vi "CreateClass.vi"(0 "ClassWriterNative":refnum<class "ClassWriterNative.lvclass">, 1 "ProjectTreePosition(String or Project Item Ref)":variant, 2 "CreateClassData":T1, 5 "error in (no error)":errorcluster, 6 "KeepLvClassRefOpen(False)":bool, 7 "HeaderToApply (take from VIRef or /use 2D-8bit header, Ignored if not wired)":variant) -> (14 "ClassWriterNative":refnum<class "ClassWriterNative.lvclass">, 15 "LVClassLibraryRefnum":refnum<vi>, 16 "TemplateVersionUsed":string, 19 "error out":errorcluster)   [LabVIEW 2012, in "ClassWriterNative.lvclass"]
uses:
  <resource>/Framework/Providers/Open_GDS/ClassProviders/Provider_LvNativeClass/ClassWriterNative_class/ClassWriterNative.lvclass
  <resource>/Framework/Providers/Open_GDS/ClassProviders/Provider_BaseClassInterface/CreateClassData.ctl
  <resource>/Framework/Providers/Open_GDS/ClassProviders/Provider_LvNativeClass/LvNativeProviderName.ctl
  <resource>/Framework/Providers/Open_GDS/ClassProviders/Provider_LvNativeClass/Templates/LvNativeTemplateNames.ctl
  <vilib>/Utility/miscctls.llb/LVPositionTypeDef.ctl
  <resource>/Framework/Providers/Open_GDS/ClassProviders/Common/LvClass_class/GDSLvCLass_ClassSettingsType.ctl
  <resource>/Framework/Providers/Open_GDS/ClassProviders/Common/LvClass_class/GDSLvClass_PlugIn.ctl
  <resource>/Framework/Providers/Open_GDS/ClassProviders/Common/LvClass_class/GDSLvClass_PlugInTypes.ctl
  <resource>/Framework/Providers/Open_GDS/ClassProviders/Provider_BaseClassInterface/ClassWriter_class/ClassWriter.lvclass
  <vilib>/Utility/lvfile.llb/NI_FileType.lvlib
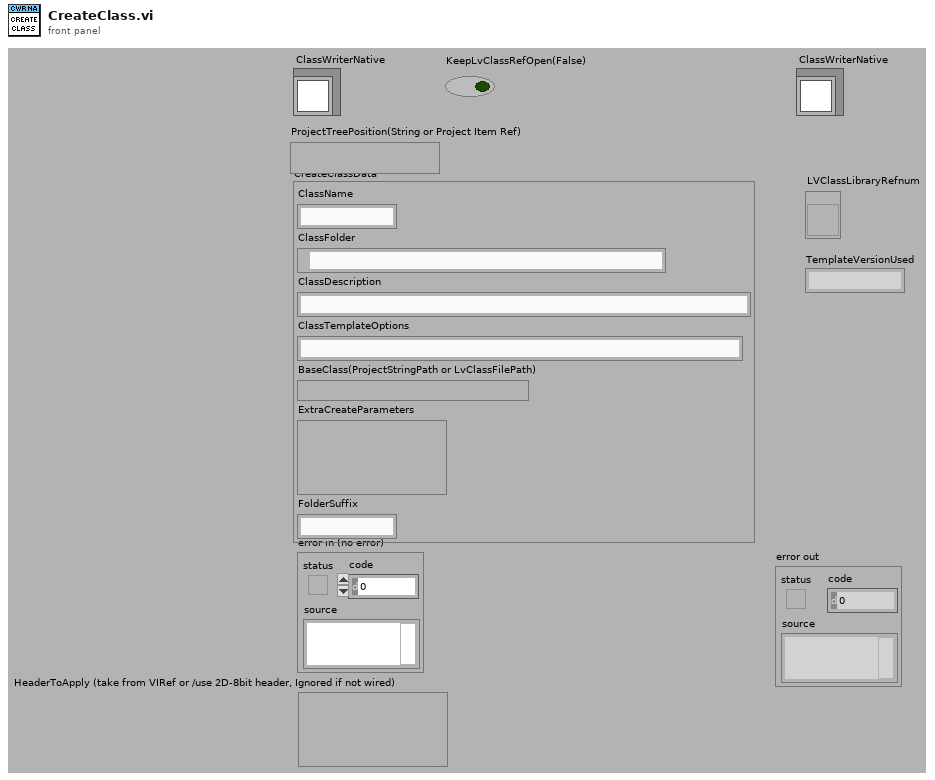
[diagram p1: front panel]
types:
  T1 = typedef "ClassWriter.lvclass/CreateClassData.ctl" = cluster{"ClassName":string, "ClassFolder":path, "ClassDescription":string, "ClassTemplateOptions":string, "BaseClass(ProjectStringPath or LvClassFilePath)":variant, "ExtraCreateParameters":variant, "FolderSuffix":string}
  T2 = cluster{"SubClass":bool, "ClassTemplateFiles":path[], "ClassName":string, "ClassFolder":path, "VIs":refnum<vi>[], "TemplateFolder":path, "ViSubDirs":string[], "TemplateName":string, "BaseClassFolder":path, "RootBaseClassFolder":path, "TemplateClass":refnum<vi>, "LvClassPath":path, "ClassRefnum":refnum<vi>, "ProjectRefnum":refnum<vi>, "LvClassFolderPath":path, "BaseClassName":string, "TemplateVersionUsed":string, "App":refnum<vi>}
  T3 = typedef "LvNativeProviderName.ctl" = enum16{"Endevo LabVIEW Native"}
  T4 = enum32{"invalid scope", "public", "private", "protected"}
  T5 = typedef "LVPositionTypeDef.ctl" = cluster{"Left":i32, "Top":i32}
  T6 = typedef "LvNativeTemplateNames.ctl" = enum16{"NativeBaseTemplate", "NativeSubTemplate", "NativeBaseTemplate_4x4x4", "NativeSubTemplate_4x4x4"}
  T7 = typedef "GDSLvCLass_ClassSettingsType.ctl" = cluster{"ClassProviderName":string, "ClassTemplateUsed":string, "ClassTemplateVersion":string, "ClassDescription":string, "PlugIns":T8[], "ConnectorPanePattern":string}
  T8 = typedef "GDSLvClass_PlugIn.ctl" = cluster{"Type":T9, "ID":string, "Version":string, "Path":path, "Name":string, "Data":variant}
  T9 = typedef "GDSLvClass_PlugInTypes.ctl" = enum16{"DesignPattern", "MethodTypes"}
  T10 = typedef "ClassWriter.lvclass/TemplateSettings.ctl" = cluster{"CommonClassTemplate":bool, "DynamicDispatch":enum8{"False", "True", "Mixed"}, "MustOverride":enum8{"False", "True", "Mixed"}, "MustCallParent":enum8{"False", "True", "Mixed"}, "OnlyNormalMethod":bool, "OnlyPublic":bool}
  T11 = typedef "Scripting_ConnectorPanePatternType.ctl" = u16
  T12 = cluster{"Major":u16, "Minor":u16, "Fix":u16, "Build":u16}
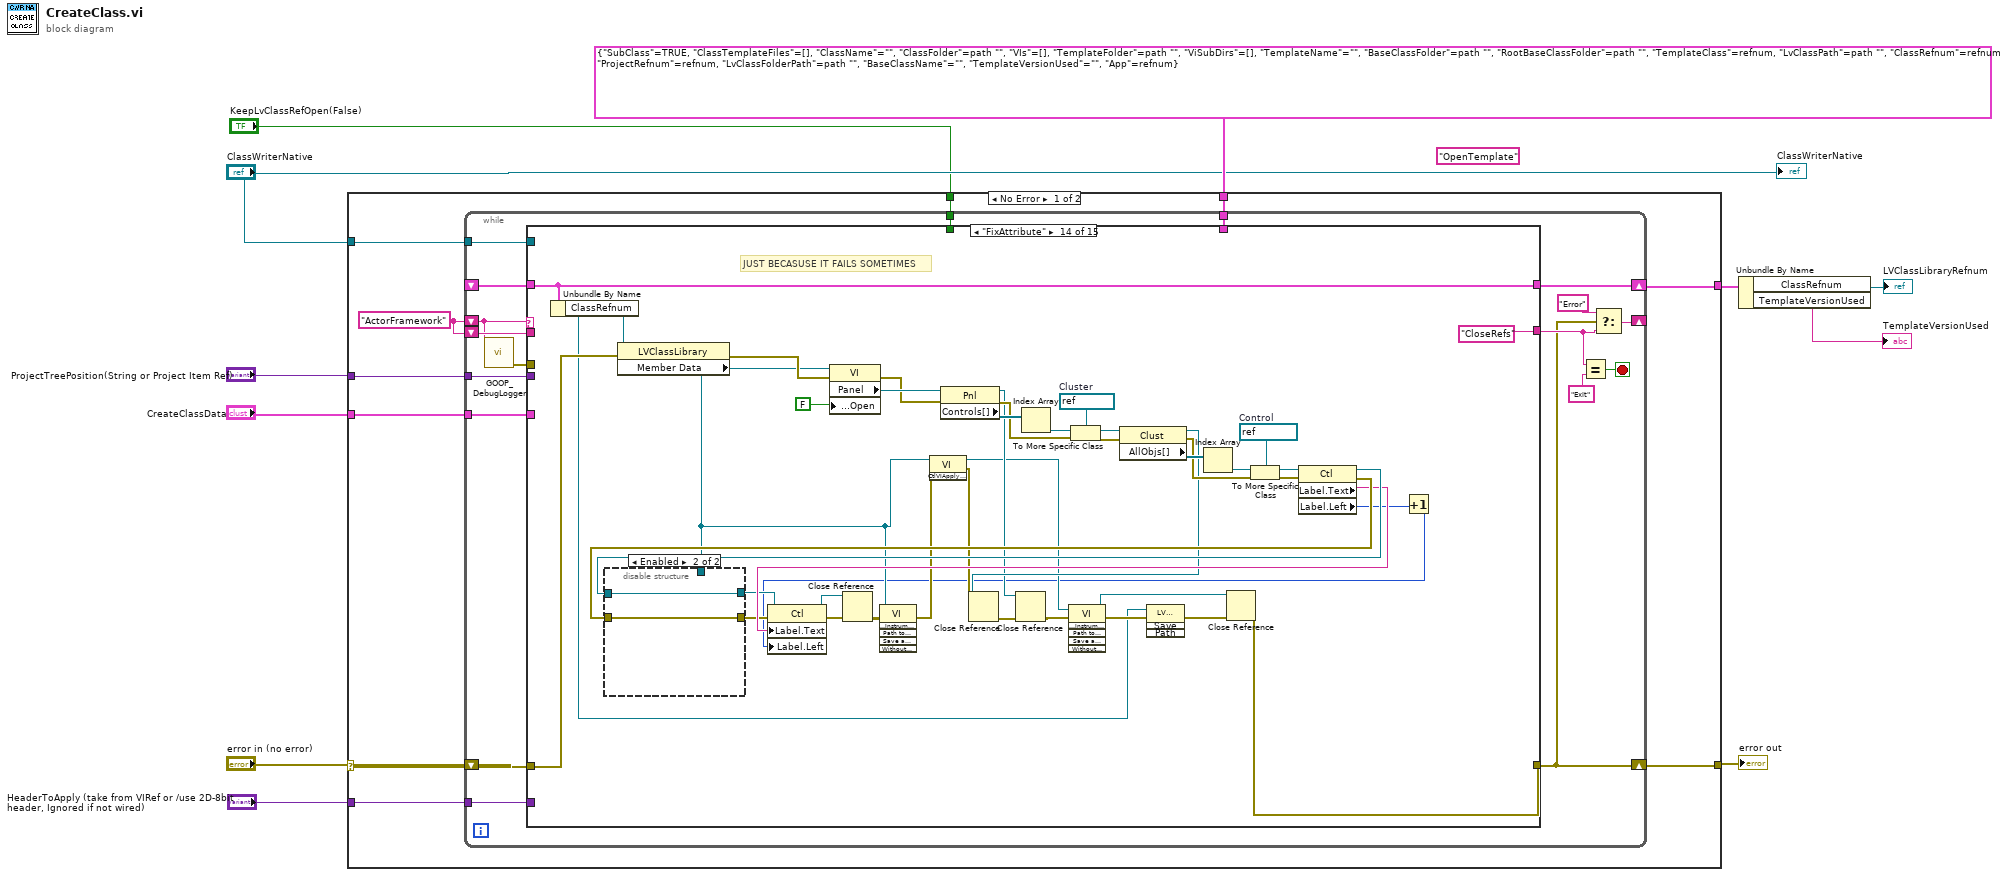
[diagram p0: block diagram]
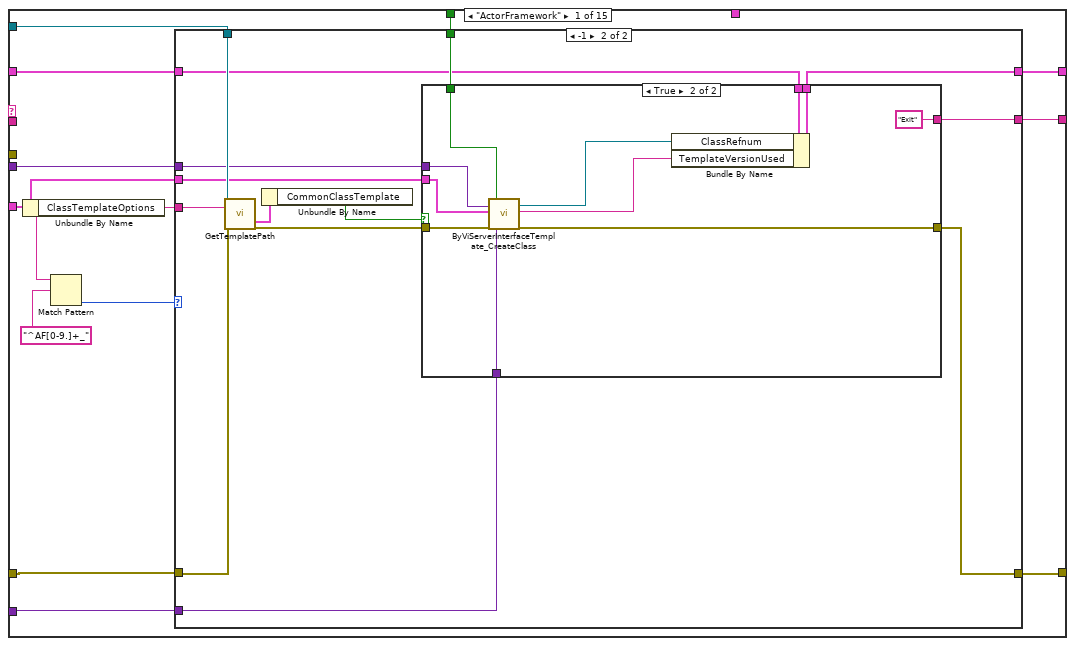
[diagram p2: hidden frame]
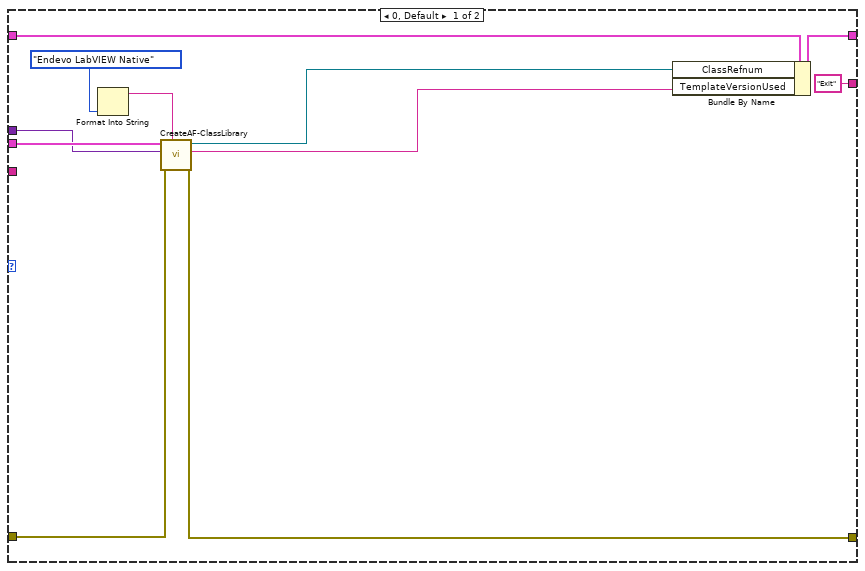
[diagram p3: hidden frame]
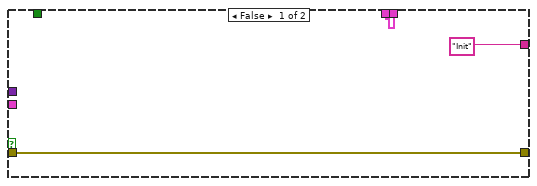
[diagram p4: hidden frame]
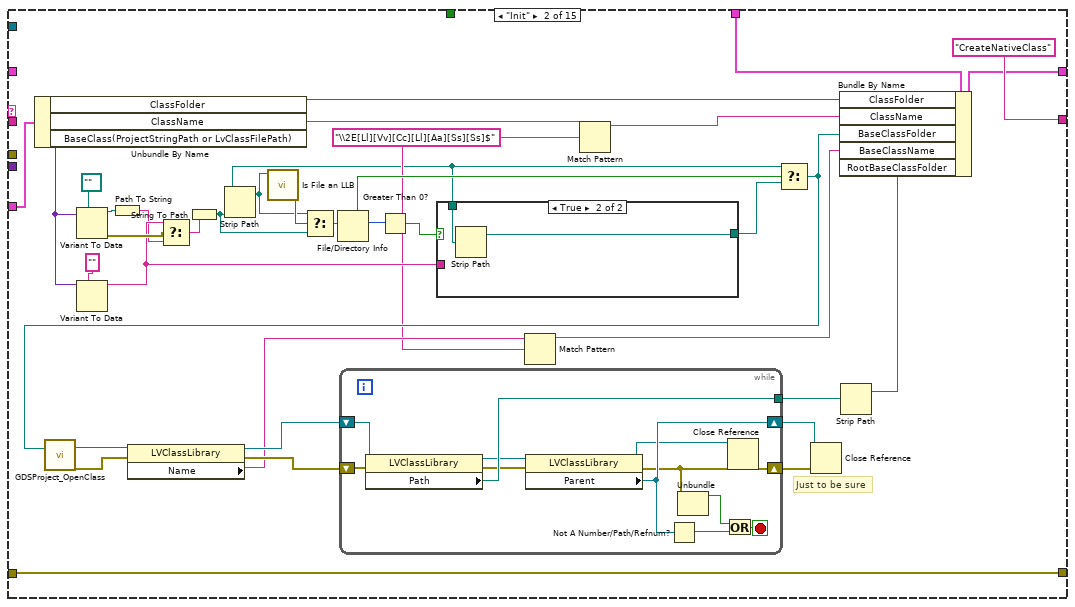
[diagram p5: hidden frame]
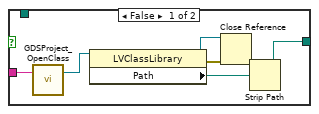
[diagram p6: hidden frame]
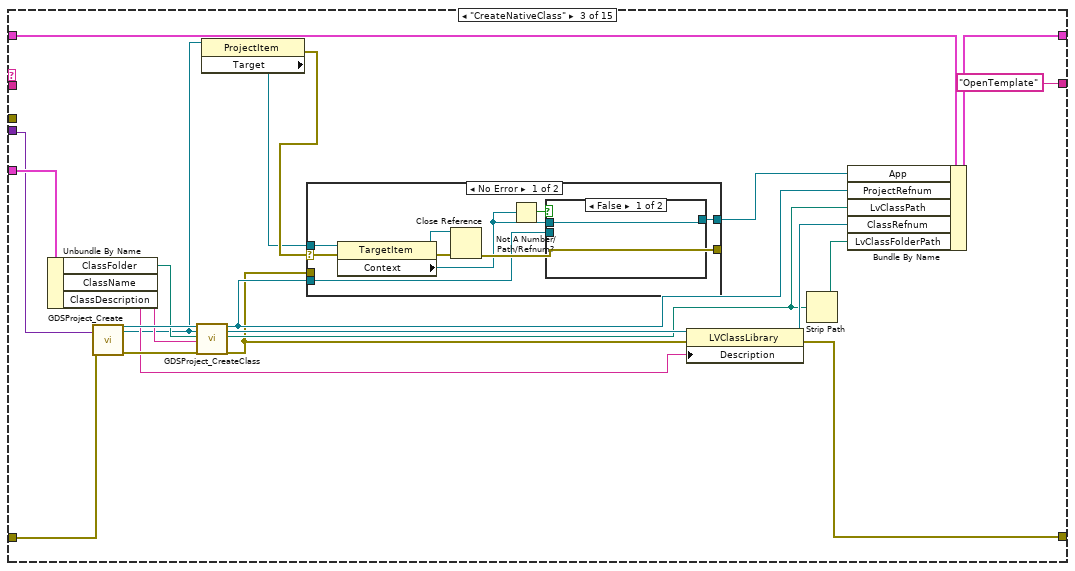
[diagram p7: hidden frame]
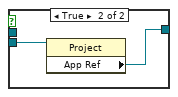
[diagram p8: hidden frame]
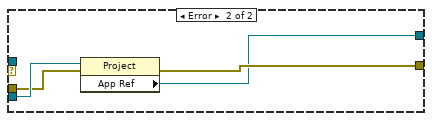
[diagram p9: hidden frame]
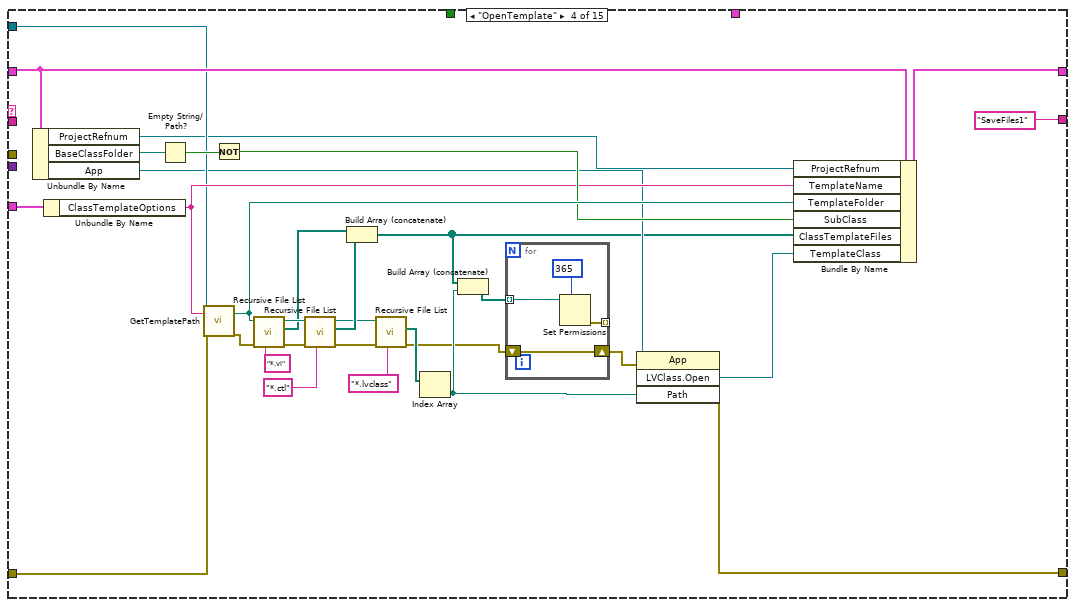
[diagram p10: hidden frame]
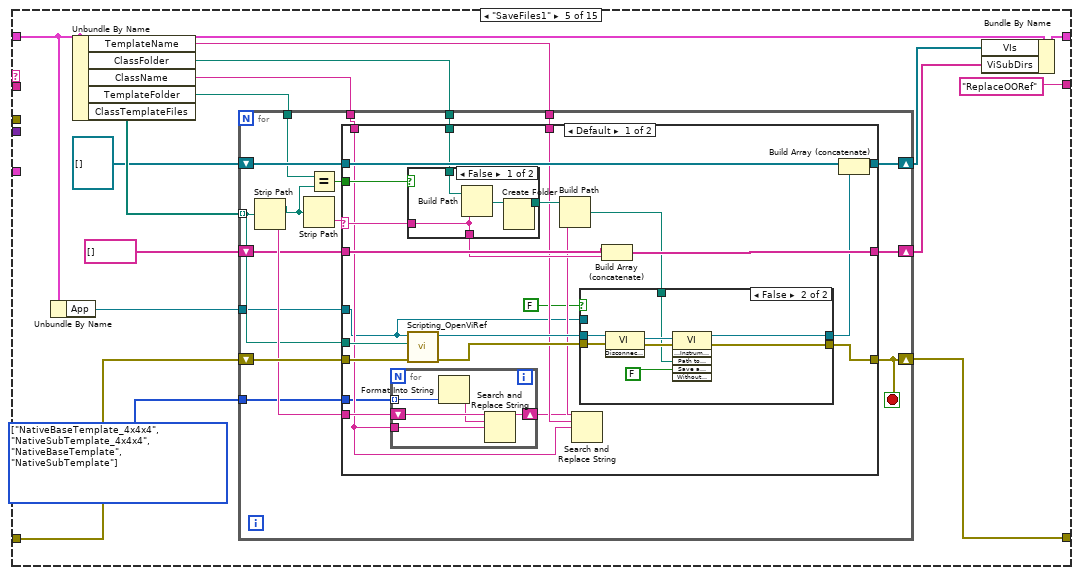
[diagram p11: hidden frame]
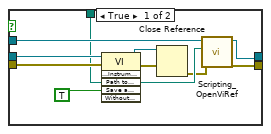
[diagram p12: hidden frame]
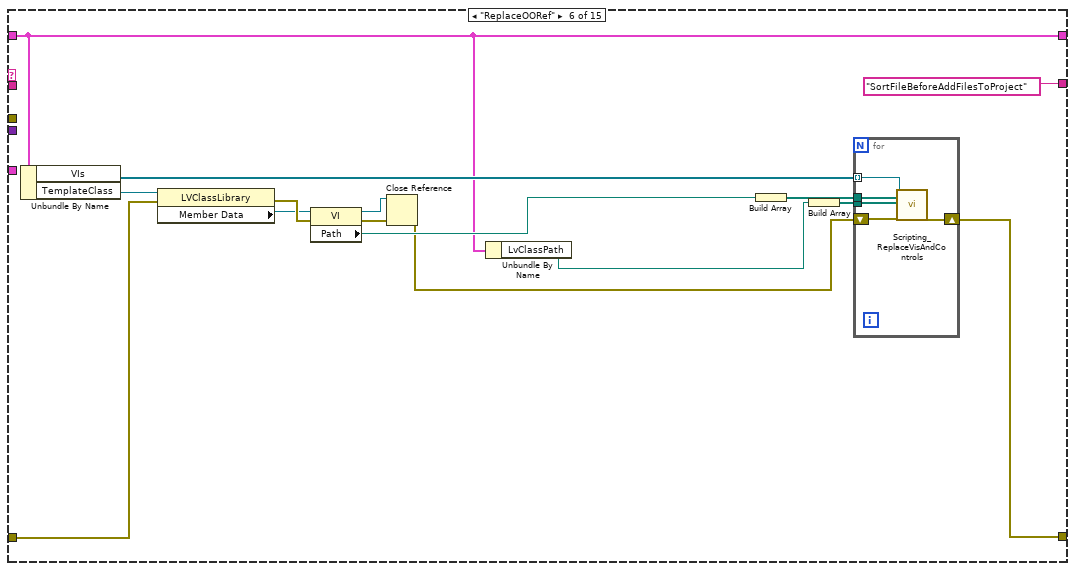
[diagram p15: hidden frame]
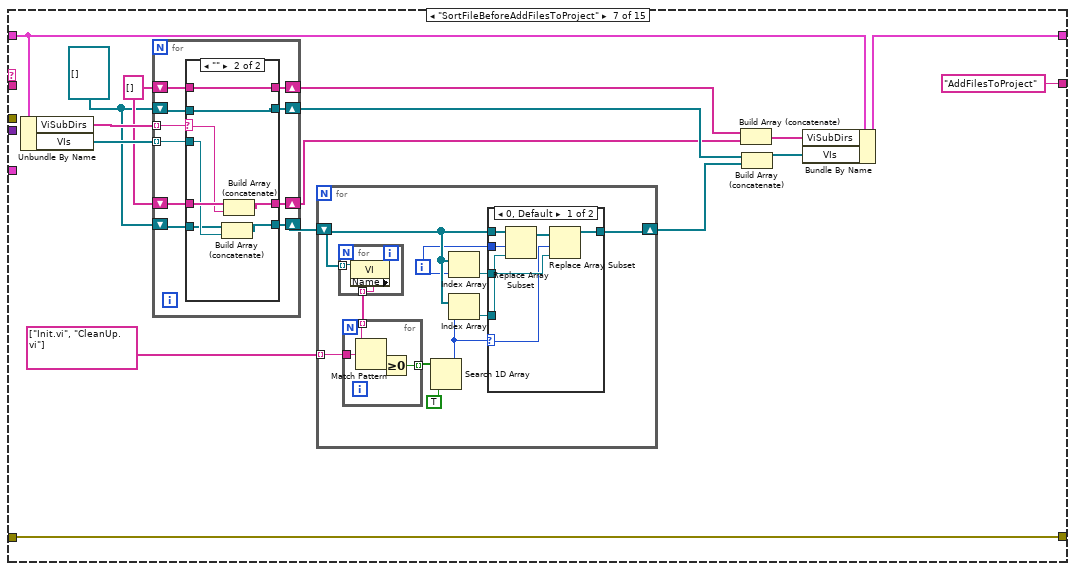
[diagram p16: hidden frame]
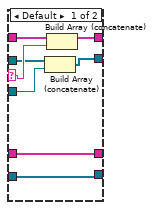
[diagram p18: hidden frame]
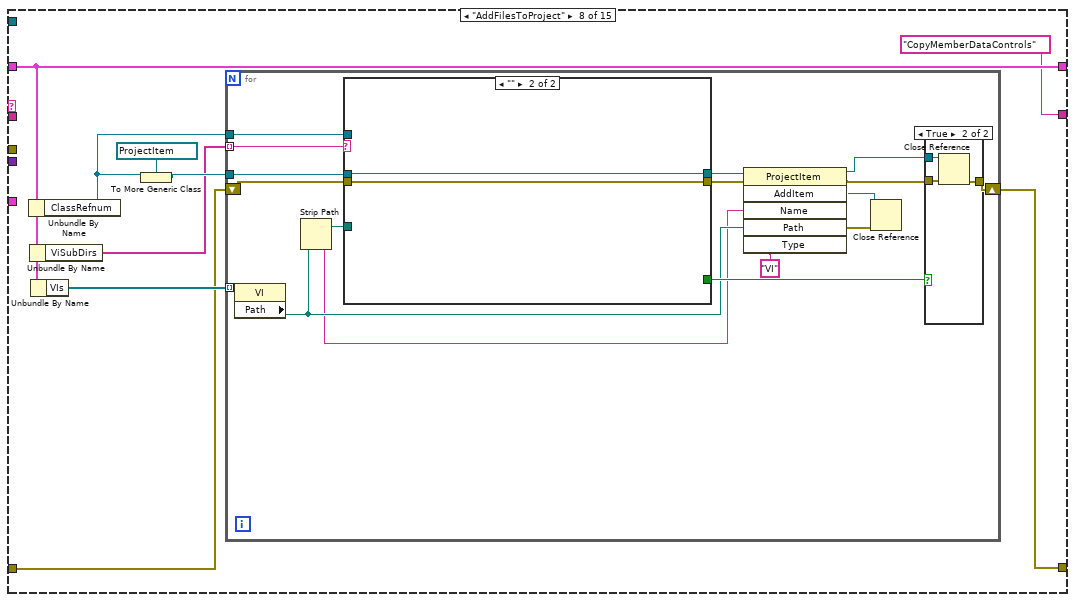
[diagram p19: hidden frame]
diagram:
  (unwired) "OpenTemplate"
  n1 = case shown="No Error" "error in (no error)" {
    selector: "error in (no error)" -> [w21 w694]
    tunnel: [w20 w694] -> w7
    tunnel: T2 {"SubClass"=TRUE, "ClassTemplateFiles"=[], "ClassName"="", "ClassFolder"=path "", "VIs"=[], "TemplateFolder"=path "", "ViSubDirs"=[], "TemplateName"="", "BaseClassFolder"=path "", "RootBaseClassFolder"=path "", "TemplateClass"=refnum, "LvClassPath"=path "", "ClassRefnum"=refnum, "ProjectRefnum"=refnum, "LvClassFolderPath"=path "", "BaseClassName"="", "TemplateVersionUsed"="", "App"=refnum} ("output cluster") -> [w19 _]
    tunnel: "ProjectTreePosition(String or Project Item Ref)" -> [w18 _]
    tunnel: "CreateClassData" -> [w17 _]
    tunnel: "ClassWriterNative" -> [w16 _]
    tunnel: "HeaderToApply (take from VIRef or /use 2D-8bit header, Ignored if not wired)" -> [w15 _]
    tunnel: "KeepLvClassRefOpen(False)" -> [w14 _]
    tunnel: [w13 _] -> w3
    frame No Error {
      w12 = "ActorFramework"
      n2 = while {
        shift-right: [w30] -> w20
        shift-left: w21 -> [w39]
        shift-right: [w34] -> _
        shift-left: w12 -> [w23]
        shift-right: [w37] -> w13
        shift-left: _ -> [w38]
        tunnel: w19 -> [w32]
        tunnel: w18 -> [w29]
        tunnel: w17 -> [w28]
        tunnel: w16 -> [w27]
        shift-left: w12 -> [w26]
        tunnel: w15 -> [w25]
        tunnel: w14 -> [w24]
        stop <- w35 stop-if-true
        n3 = call <resource>:"GOOP_DebugLogger.vi"("State"=w23) -> ("error out"=w22:errorcluster)  [unwired: 10 in]
        n4 = case shown="\"FixAttribute\"" w23 {
          selector: w23 -> [_ _ _ _ _ _ _ _ _ _ _ _ _ _ w669]
          tunnel: w38 -> [w50 _ w156 w201 w224 w310 w342 w397 w502 w517 w536 w557 w566 w644 w666]
          tunnel: [w47 w124 w155 w215 w230 w310 w341 w397 w502 w517 w536 w557 w565 w644 w666] -> w37
          tunnel: w39 -> [w48 w127 w158 w195 w221 w316 w340 w395 w462 w508 w529 w555 w573 w622 w675]
          tunnel: [w45 w127 w154 w190 w220 w321 w340 w402 w452 w505 w540 w549 w590 w623 w668] -> w30
          tunnel: [w46 "CreateNativeClass" "OpenTemplate" "SaveFiles1" "ReplaceOORef" "SortFileBeforeAddFilesToProject" "AddFilesToProject" "CopyMemberDataControls" "UpdateIcons" w519 "AddFolders" "SetClassProperties" "FixAttribute" "CloseRefs" "Exit"] -> w31
          tunnel: w32 -> [_ w112 _ _ _ _ _ _ _ _ _ _ _ _ _]
          tunnel: w29 -> [w44 _ w157 _ _ _ _ _ _ _ _ _ _ _ _]
          tunnel: w28 -> [w49 w111 w159 w197 _ _ _ _ _ _ _ _ w587 _ _]
          tunnel: w27 -> [w42 _ _ w198 _ _ _ _ _ w504 w531 _ _ _ _]
          tunnel: w26 -> [_ _ _ _ _ _ _ _ _ _ _ _ _ _ w667]
          tunnel: w25 -> [w40 _ _ _ _ _ _ _ _ w513 _ _ _ _ _]
          tunnel: w24 -> [w41 _ _ _ _ _ _ _ _ _ _ _ _ _ w664]
          tunnel: w22 -> [_ _ _ _ _ _ _ _ _ _ _ _ _ _ _]
          frame "ActorFramework" {
            n5 = Unbundle By Name(w49) -> ("ClassTemplateOptions"=w43:string)
            n6 = Match Pattern(string=w43, regular expression="^AF[0-9.]+_") -> (offset past match=w52:i32)  [unwired: 1 in, 3 out]
            n7 = case shown="-1" w52 {
              tunnel: w50 -> [w63 w67]
              tunnel: [w62 w66] -> w47
              tunnel: ["Exit" w74] -> w46
              tunnel: w49 -> [w60 w69]
              tunnel: w48 -> [w59 w75]
              tunnel: [w58 w72] -> w45
              tunnel: w44 -> [w53 w70]
              tunnel: w43 -> [_ w77]
              tunnel: w42 -> [_ w76]
              tunnel: w41 -> [_ w71]
              tunnel: w40 -> [_ w68]
              frame 0, Default {
                n8 = Format Into String(LvNativeProviderName."Endevo LabVIEW Native" ("ProviderName")) -> (resulting string=w57:string)  [unwired: 3 in, 1 out]
                n9 = call <resource>:"CreateAF-ClassLibrary.vi"("Providername"=w57, "error in (no error)"=w59, "ProjectTreePosition(String or Project Item Ref)"=w53, "CreateClassData"=w60) -> ("error out"=w58:errorcluster, "TemplateVersionUsed"=w55:string, "LVClassLibraryRefnum"=w56:refnum<vi>)  [unwired: 5 in]
                n10 = Bundle By Name(cluster=w63, "ClassRefnum"=w56, "TemplateVersionUsed"=w55) -> (w62:T2)
              }
              frame -1 {
                n11 = call-dynamic "GetTemplatePath.vi"("reference in"=w76, "ClassTemplateSubDirectory"=w77, "error in (no error)"=w75) -> ("TemplateSettings"=w65:T10, "error out"=w73:errorcluster)  [unwired: 12 in, 3 out]
                n12 = Unbundle By Name(w65) -> ("CommonClassTemplate"=w64:bool)
                n13 = case shown="True" w64 {
                  tunnel: ["Init" "Exit"] -> w74
                  tunnel: w73 -> [w79 w90]
                  tunnel: [w79 w89] -> w72
                  tunnel: w71 -> [_ w88]
                  tunnel: w70 -> [_ w87]
                  tunnel: w69 -> [_ w86]
                  tunnel: w68 -> [_ w85]
                  tunnel: w67 -> [w78 w84]
                  tunnel: [w78 w83] -> w66
                  frame False {
                  }
                  frame True {
                    n14 = call <resource>:"ByViServerInterfaceTemplate_CreateClass.vi"("ProjectTreePosition(String or Project Item Ref)"=w87, "CreateClassData"=w86, "error in (no error)"=w90, "KeepLvClassRefOpen(False)"=w88, "HeaderToApply (take from VIRef or /use 2D-8bit header, Ignored if not wired)"=w85) -> ("LVClassLibraryRefnum"=w82:refnum<vi>, "TemplateVersionUsed"=w81:string, "error out"=w89:errorcluster)  [unwired: 12 in]
                    n15 = Bundle By Name(cluster=w84, "ClassRefnum"=w82, "TemplateVersionUsed"=w81) -> (w83:T2)
                  }
                }
              }
            }
          }
          frame "Init" {
            w97 = "\\2E[Ll][Vv][Cc][Ll][Aa][Ss][Ss]$" ("regular expression")
            # "Just to be sure"
            n16 = Unbundle By Name(w111) -> ("ClassFolder"=w110:path, "ClassName"=w109:string, "BaseClass(ProjectStringPath or LvClassFilePath)"=w108:variant)
            n17 = Variant To Data(type=path "" ("path"), Variant=w108) -> (data=w114:path, error out=w118:errorcluster)  [unwired: 1 in]
            n18 = Variant To Data(type="" ("regular expression"), Variant=w108) -> (data=w115:string)  [unwired: 1 in, 1 out]
            n19 = Path To String(path=w114) -> (string=w113:string)
            n20 = Select(t=w115, s=w118, f=w113) -> (s? t:f=w117:string)
            n21 = String To Path(string=w117) -> (path=w93:path)
            n22 = Strip Path(path=w93) -> (stripped path=w94:path)  [unwired: 1 out]
            n23 = call <vilib>:"Is File an LLB.vi"("path"=w94) -> ("Is LLB?"=w95:bool)  [unwired: 9 in, 1 out]
            n24 = Select(t=w94, s=w95, f=w93) -> (s? t:f=w92:path)
            n25 = File/Directory Info(path=w92) -> (directory=w122:bool, size=w121:i64)  [unwired: 1 in, 5 out]
            n26 = Greater Than 0?(x=w121) -> (x > 0?=w119:bool)
            n27 = case shown="True" w119 {
              tunnel: w93 -> [_ w146]
              tunnel: [w143 w145] -> w120
              tunnel: w115 -> [w144 _]
              frame False {
                n28 = call <resource>:"GDSProject_OpenClass.vi"("ClassPath(FilePath/ProjectTreePath/LvCLassRef)"=w144) -> ("LVClass.Open"=w141:refnum<vi>)  [unwired: 16 in, 2 out]
                n29 = property class="LVClassLibrary"(reference=w141) -> (reference out=w139:refnum<vi>, error out=w140:errorcluster, "Path"=w142:path)  [unwired: 1 in]
                n30 = Close Reference(reference=w139, error in (no error)=w140) -> ()  [unwired: 1 out]
                n31 = Strip Path(path=w142) -> (stripped path=w143:path)  [unwired: 1 out]
              }
              frame True {
                n32 = Strip Path(path=w146) -> (stripped path=w145:path)  [unwired: 1 out]
              }
            }
            n33 = Match Pattern(string=w109, regular expression=w97) -> (before substring=w125:string)  [unwired: 1 in, 3 out]
            n34 = Select(t=w93, s=w122, f=w120) -> (s? t:f=w107:path)
            n35 = call <resource>:"GDSProject_OpenClass.vi"("ClassPath(FilePath/ProjectTreePath/LvCLassRef)"=w107) -> ("LVClass.Open"=w100:refnum<vi>, "error out"=w102:errorcluster)  [unwired: 16 in, 1 out]
            n36 = property class="LVClassLibrary"(reference=w100, error in=w102) -> (reference out=w99:refnum<vi>, error out=w101:errorcluster, "Name"=w98:string)
            n37 = while {
              shift-right: [w135] -> w106
              shift-left: w101 -> [w130]
              shift-right: [w136] -> w105
              shift-left: w99 -> [w138]
              tunnel: [w137] -> w104
              stop <- w132 stop-if-true
              n38 = property class="LVClassLibrary"(reference=w138, error in=w130) -> (reference out=w128:refnum<vi>, error out=w129:errorcluster, "Path"=w137:path)
              n39 = property class="LVClassLibrary"(reference=w128, error in=w129) -> (reference out=w131:refnum<vi>, error out=w135:errorcluster, "Parent"=w136:refnum<vi>)
              n40 = Not A Number/Path/Refnum?(number/path/refnum=w136) -> (NaN/Path/Refnum?=w133:bool)
              n41 = Unbundle(w135) -> ("status"=w134:bool)  [unwired: 2 out]
              n42 = Or(x=w134, y=w133) -> (x .or. y?=w132:bool)
              n43 = Close Reference(reference=w131) -> ()  [unwired: 1 in, 1 out]
            }
            n44 = Match Pattern(string=w98, regular expression=w97) -> (before substring=w96:string)  [unwired: 1 in, 3 out]
            n45 = Close Reference(reference=w105, error in (no error)=w106) -> ()  [unwired: 1 out]
            n46 = Strip Path(path=w104) -> (stripped path=w103:path)  [unwired: 1 out]
            n47 = Bundle By Name(cluster=w112, "ClassFolder"=w110, "ClassName"=w125, "BaseClassFolder"=w107, "BaseClassName"=w96, "RootBaseClassFolder"=w103) -> (w124:T2)
          }
          frame "CreateNativeClass" {
            n48 = Unbundle By Name(w159) -> ("ClassFolder"=w163:path, "ClassName"=w164:string, "ClassDescription"=w160:string)
            n49 = call <resource>:"GDSProject_Create.vi"("ProjectTreePosition(String or Project Item Ref)"=w157, "error in (no error)"=w158) -> ("Project Refnum"=w167:refnum<vi>, "Project Item"=w153:refnum<vi>, "error out"=w166:errorcluster)  [unwired: 15 in]
            n50 = call <resource>:"GDSProject_CreateClass.vi"("Project Refnum In"=w167, "Project Item To Create Class Below(Use MyComputer if not wired)"=w153, "ClassFolder"=w163, "ClassName"=w164, "error in (no error)"=w166) -> ("Project Refnum Out"=w149:refnum<vi>, "Class Refnum Out"=w162:refnum<vi>, "ClassPathOut"=w150:path, "error out"=w148:errorcluster)  [unwired: 11 in]
            n51 = property class="ProjectItem"(reference=w153) -> (error out=w152:errorcluster, "Target"=w151:refnum<vi>)  [unwired: 1 in, 1 out]
            n52 = case shown="No Error" w152 {
              selector: w152 -> [w173 _]
              tunnel: w151 -> [w177 _]
              tunnel: [w174 w182] -> _
              tunnel: w148 -> [_ w183]
              tunnel: [w170 w181] -> w147
              tunnel: w149 -> [w169 w184]
              frame No Error {
                n53 = property class="TargetItem"(reference=w177, error in=w173) -> (reference out=w175:refnum<vi>, error out=w176:errorcluster, "Context"=w171:refnum<vi>)
                n54 = Close Reference(reference=w175, error in (no error)=w176) -> (error out=w174:errorcluster)
                n55 = Not A Number/Path/Refnum?(number/path/refnum=w171) -> (NaN/Path/Refnum?=w172:bool)
                n56 = case shown="False" w172 {
                  tunnel: [w178 w179] -> w170
                  tunnel: w169 -> [_ w180]
                  tunnel: w171 -> [w178 _]
                  frame False {
                  }
                  frame True {
                    n57 = property class="Project"(reference=w180) -> ("App Ref"=w179:refnum<vi>)  [unwired: 1 in, 2 out]
                  }
                }
              }
              frame Error {
                n58 = property class="Project"(reference=w184, error in=w183) -> (error out=w182:errorcluster, "App Ref"=w181:refnum<vi>)  [unwired: 1 out]
              }
            }
            n59 = property class="LVClassLibrary"(reference=w162, error in=w148, "Description"=w160) -> (reference out=w161:refnum<vi>, error out=w154:errorcluster)
            n60 = Strip Path(path=w150) -> (stripped path=w165:path)  [unwired: 1 out]
            n61 = Bundle By Name(cluster=w156, "App"=w147, "ProjectRefnum"=w149, "LvClassPath"=w150, "ClassRefnum"=w161, "LvClassFolderPath"=w165) -> (w155:T2)
          }
          frame "OpenTemplate" {
            n62 = Unbundle By Name(w201) -> ("ProjectRefnum"=w192:refnum<vi>, "BaseClassFolder"=w203:path, "App"=w191:refnum<vi>)
            n63 = Unbundle By Name(w197) -> ("ClassTemplateOptions"=w199:string)
            n64 = Empty String/Path?(string/path=w203) -> (empty?=w202:bool)
            n65 = call-dynamic "GetTemplatePath.vi"("reference in"=w198, "ClassTemplateSubDirectory"=w199, "error in (no error)"=w195) -> ("FolderPathOut"=w204:path, "error out"=w194:errorcluster)  [unwired: 12 in, 3 out]
            n66 = Not(x=w202) -> (.not. x?=w200:bool)
            n67 = call <vilib>:"Recursive File List.vi"("pattern"="*.vi", "error in (no error)"=w194, "Folder Path"=w204) -> ("error out"=w209:errorcluster, "All Files in Dir"=w211:path[], "dup Folder Path"=w213:path)  [unwired: 4 in, 2 out]
            n68 = call <vilib>:"Recursive File List.vi"("pattern"="*.ctl", "error in (no error)"=w209, "Folder Path"=w213) -> ("error out"=w208:errorcluster, "All Files in Dir"=w210:path[], "dup Folder Path"=w207:path)  [unwired: 4 in, 2 out]
            n69 = Build Array (concatenate)(w211, w210) -> (w189:path[])
            n70 = call <vilib>:"Recursive File List.vi"("pattern"="*.lvclass", "error in (no error)"=w208, "Folder Path"=w207) -> ("error out"=w187:errorcluster, "All Files in Dir"=w205:path[])  [unwired: 4 in, 3 out]
            n71 = Index Array(array=w205) -> (element=w188:path)  [unwired: 1 in]
            n72 = Build Array (concatenate)(w189, w188) -> (w185:path[])
            n73 = for {
              tunnel: w185 -> [w218] mode=indexing
              shift-right: [w219] -> w186
              shift-left: w187 -> [w219]
              tunnel: [w216] -> _ mode=indexing
              n74 = Set Permissions(7:i16 365 ("permissions"), 11:w218) -> (0:w216:errorcluster)  [unwired: 3 in, 1 out]
            }
            n75 = invoke class="App" method="LVClass.Open"(reference=w191, error in=w186, "Path"=w188) -> (error out=w190:errorcluster, "LVClass.Open"=w193:refnum<vi>)  [unwired: 1 in, 2 out]
            n76 = Bundle By Name(cluster=w201, "ProjectRefnum"=w192, "TemplateName"=w199, "TemplateFolder"=w204, "SubClass"=w200, "ClassTemplateFiles"=w189, "TemplateClass"=w193) -> (w215:T2)
          }
          frame "SaveFiles1" {
            w223 = T6[] [enum."NativeBaseTemplate_4x4x4", enum."NativeSubTemplate_4x4x4", enum."NativeBaseTemplate", enum."NativeSubTemplate"] items=["NativeBaseTemplate", "NativeSubTemplate", "NativeBaseTemplate_4x4x4", "NativeSubTemplate_4x4x4"]
            n77 = Unbundle By Name(w224) -> ("App"=w222:refnum<vi>)
            n78 = Unbundle By Name(w224) -> ("TemplateName"=w225:string, "ClassFolder"=w234:path, "ClassName"=w233:string, "TemplateFolder"=w228:path, "ClassTemplateFiles"=w235:path[])
            n79 = for {
              tunnel: w235 -> [w241] mode=indexing
              shift-right: [w246] -> w231
              shift-left: refnum<vi>[] [] -> [w247]
              shift-right: [w236] -> w220
              shift-left: w221 -> [w251]
              tunnel: w234 -> [w250]
              tunnel: w233 -> [w248]
              tunnel: w228 -> [w243]
              shift-right: [w242] -> w226
              shift-left: string[] [] -> [w240]
              tunnel: w222 -> [w239]
              tunnel: w225 -> [w238]
              tunnel: w223 -> [w237]
              stop <- w236 stop-if-true
              n80 = Strip Path(path=w241) -> (stripped path=w245:path, name=w249:string)
              n81 = Strip Path(path=w245) -> (name=w252:string)  [unwired: 1 out]
              n82 = Equal?(x=w243, y=w245) -> (x = y?=w244:bool)
              n83 = case shown="Default" w252 {
                selector: w252 -> [w270 _]
                tunnel: w241 -> [w276 _]
                tunnel: w251 -> [w275 w306]
                tunnel: [w262 w306] -> w236
                tunnel: w250 -> [w271 _]
                tunnel: w249 -> [w274 _]
                tunnel: w248 -> [w257 _]
                tunnel: w247 -> [w273 w307]
                tunnel: [w272 w307] -> w246
                tunnel: w244 -> [w268 _]
                tunnel: [w266 w305] -> w242
                tunnel: w240 -> [w267 w305]
                tunnel: w239 -> [w253 _]
                tunnel: w238 -> [w258 _]
                tunnel: w237 -> [w255 _]
                frame Default {
                  n84 = for {
                    tunnel: w257 -> [w297]
                    shift-right: [w299] -> w256
                    shift-left: w274 -> [w298]
                    tunnel: w255 -> [w296] mode=indexing
                    n85 = Format Into String(w296) -> (resulting string=w295:string)  [unwired: 3 in, 1 out]
                    n86 = Search and Replace String(input string=w298, search string=w295, replace string=w297) -> (result string=w299:string)  [unwired: 5 in, 3 out]
                  }
                  n87 = case shown="False" w268 {
                    tunnel: w271 -> [w303 w304]
                    tunnel: w270 -> [w300 _]
                    tunnel: [w301 w304] -> w269
                    tunnel: [w300 _] -> w265
                    frame False {
                      n88 = Build Path(base path=w303, name or relative path=w300) -> (appended path=w302:path)
                      n89 = Create Folder(path (use dialog)=w302) -> (created path=w301:path)  [unwired: 2 in, 2 out]
                    }
                    frame True {
                    }
                  }
                  n90 = call <resource>:"Scripting_OpenViRef.vi"("error in"=w275, "ViPath/ViName"=w276, "AppRef"=w253) -> ("error out"=w264:errorcluster, "vi reference"=w263:refnum<vi>)  [unwired: 7 in]
                  n91 = Search and Replace String(input string=w256, search string=w258, replace string=w257) -> (result string=w259:string)  [unwired: 5 in, 3 out]
                  n92 = Build Path(base path=w269, name or relative path=w259) -> (appended path=w260:path)
                  n93 = case shown="False" FALSE {
                    tunnel: w264 -> [w285 w294]
                    tunnel: w263 -> [w286 w293]
                    tunnel: [w281 w290] -> w262
                    tunnel: [w280 w289] -> w261
                    tunnel: w260 -> [w282 w288]
                    tunnel: w253 -> [w283 _]
                    frame True {
                      n94 = invoke class="VI" method="Save.Instrument"(reference=w286, error in=w285, "Path to saved file"=w282, "Save a Copy"=TRUE) -> (reference out=w278:refnum<vi>, error out=w279:errorcluster)  [unwired: 2 in, 4 out]
                      n95 = Close Reference(reference=w278, error in (no error)=w279) -> (error out=w277:errorcluster)
                      n96 = call <resource>:"Scripting_OpenViRef.vi"("error in"=w277, "ViPath/ViName"=w282, "AppRef"=w283) -> ("error out"=w281:errorcluster, "vi reference"=w280:refnum<vi>)  [unwired: 7 in]
                    }
                    frame False {
                      n97 = invoke class="VI" method="DisconnectFromLibrary"(reference=w293, error in=w294) -> (reference out=w292:refnum<vi>, error out=w291:errorcluster)  [unwired: 1 in, 1 out]
                      n98 = invoke class="VI" method="Save.Instrument"(reference=w292, error in=w291, "Path to saved file"=w288, "Save a Copy"=FALSE) -> (reference out=w289:refnum<vi>, error out=w290:errorcluster)  [unwired: 2 in, 4 out]
                    }
                  }
                  n99 = Build Array (concatenate)(w267, w265) -> (w266:string[])
                  n100 = Build Array (concatenate)(w273, w261) -> (w272:refnum<vi>[])
                }
                frame "methods" {
                }
              }
            }
            n101 = Bundle By Name(cluster=w224, "VIs"=w231, "ViSubDirs"=w226) -> (w230:T2)
          }
          frame "ReplaceOORef" {
            n102 = Unbundle By Name(w310) -> ("VIs"=w322:refnum<vi>[], "TemplateClass"=w317:refnum<vi>)
            n103 = property class="LVClassLibrary"(reference=w317, error in=w316) -> (error out=w319:errorcluster, "Member Data"=w318:refnum<vi>)  [unwired: 1 out]
            n104 = property class="VI"(reference=w318, error in=w319) -> (reference out=w311:refnum<vi>, error out=w312:errorcluster, "Path"=w315:path)
            n105 = Close Reference(reference=w311, error in (no error)=w312) -> (error out=w308:errorcluster)
            n106 = Unbundle By Name(w310) -> ("LvClassPath"=w309:path)
            n107 = Build Array(w315) -> (w314:path[])
            n108 = Build Array(w309) -> (w313:path[])
            n109 = for {
              tunnel: w322 -> [w325] mode=indexing
              shift-right: [w326] -> w321
              shift-left: w308 -> [w327]
              tunnel: w313 -> [w324]
              tunnel: w314 -> [w323]
              n110 = call <resource>:"Scripting_ReplaceVisAndControls.vi"("ViRef"=w325, "OldVIsAndControls"=w323, "NewVIsAndControls"=w324, "error in (no error)"=w327) -> ("error out"=w326:errorcluster)  [unwired: 14 in, 1 out]
            }
          }
          frame "SortFileBeforeAddFilesToProject" {
            w332 = refnum<vi>[] []
            w333 = string[] []
            n111 = Unbundle By Name(w342) -> ("ViSubDirs"=w339:string[], "VIs"=w338:refnum<vi>[])
            n112 = for {
              tunnel: w339 -> [w377] mode=indexing
              tunnel: w338 -> [w372] mode=indexing
              shift-right: [w375] -> w337
              shift-left: w333 -> [w376]
              shift-right: [w373] -> w334
              shift-left: w332 -> [w374]
              shift-right: [w369] -> w331
              shift-left: w333 -> [w368]
              shift-right: [w371] -> w330
              shift-left: w332 -> [w370]
              n113 = case shown="\"\"" w377 {
                selector: w377 -> [w383 w389]
                tunnel: w376 -> [w385 w393]
                tunnel: [w384 w393] -> w375
                tunnel: w374 -> [w382 w392]
                tunnel: [w381 w392] -> w373
                tunnel: w372 -> [w380 w388]
                tunnel: w368 -> [w379 w391]
                tunnel: [w379 w390] -> w369
                tunnel: w370 -> [w378 w387]
                tunnel: [w378 w386] -> w371
                frame Default {
                  n114 = Build Array (concatenate)(w382, w380) -> (w381:refnum<vi>[])
                  n115 = Build Array (concatenate)(w385, w383) -> (w384:string[])
                }
                frame "" {
                  n116 = Build Array (concatenate)(w387, w388) -> (w386:refnum<vi>[])
                  n117 = Build Array (concatenate)(w391, w389) -> (w390:string[])
                }
              }
            }
            n118 = for {
              shift-right: [w349] -> w328
              shift-left: w330 -> [w353]
              tunnel: string[] ["Init.vi", "CleanUp.vi"] -> [w347] mode=indexing
              i -> [w352]
              n119 = for {
                tunnel: w353 -> [w367] mode=indexing
                tunnel: [w366] -> w348 mode=indexing
                n120 = property class="VI"(reference=w367) -> ("Name"=w366:string)  [unwired: 1 in, 2 out]
              }
              n121 = for {
                tunnel: w348 -> [w357] mode=indexing
                tunnel: w347 -> [w356]
                tunnel: [w354] -> w346 mode=indexing
                n122 = Match Pattern(string=w357, regular expression=w356) -> (offset past match=w355:i32)  [unwired: 1 in, 3 out]
                n123 = Greater Or Equal To 0?(x=w355) -> (x >= 0?=w354:bool)
              }
              n124 = Search 1D Array(1D array=w346, element=TRUE) -> (index of element=w344:i32)  [unwired: 1 in]
              n125 = Index Array(array=w353, index=w352) -> (element=w350:refnum<vi>)
              n126 = Index Array(array=w353, index=w344) -> (element=w351:refnum<vi>)
              n127 = case shown="0, Default" w344 {
                selector: w344 -> [w359 _]
                tunnel: w353 -> [w364 w365]
                tunnel: w352 -> [w363 _]
                tunnel: w351 -> [w362 _]
                tunnel: w350 -> [w360 _]
                tunnel: [w358 w365] -> w349
                frame 0, Default {
                  n128 = Replace Array Subset(array=w364, new element=w362, index=w363) -> (w361:refnum<vi>[])
                  n129 = Replace Array Subset(array=w361, new element=w360, index=w359) -> (w358:refnum<vi>[])
                }
                frame -1 {
                }
              }
            }
            n130 = Build Array (concatenate)(w337, w331) -> (w336:string[])
            n131 = Build Array (concatenate)(w334, w328) -> (w335:refnum<vi>[])
            n132 = Bundle By Name(cluster=w342, "ViSubDirs"=w336, "VIs"=w335) -> (w341:T2)
          }
          frame "AddFilesToProject" {
            n133 = Unbundle By Name(w397) -> ("ClassRefnum"=w396:refnum<vi>)
            n134 = Unbundle By Name(w397) -> ("ViSubDirs"=w399:string[])
            n135 = Unbundle By Name(w397) -> ("VIs"=w398:refnum<vi>[])
            n136 = To More Generic Class(target class=refnum<vi> refnum ("AddItem"), reference=w396) -> (generic class reference=w400:refnum<vi>)
            n137 = for {
              tunnel: w399 -> [w407] mode=indexing
              tunnel: w400 -> [w416]
              shift-right: [w412] -> w402
              shift-left: w395 -> [w414]
              tunnel: w396 -> [w406]
              tunnel: w398 -> [w408] mode=indexing
              n138 = property class="VI"(reference=w408) -> ("Path"=w409:path)  [unwired: 1 in, 2 out]
              n139 = Strip Path(path=w409) -> (stripped path=w417:path, name=w405:string)
              n140 = case shown="\"\"" w407 {
                selector: w407 -> [w425 _]
                tunnel: w416 -> [w431 w450]
                tunnel: [w428 w450] -> w415
                tunnel: w414 -> [w430 w449]
                tunnel: [w426 w449] -> w418
                tunnel: w417 -> [_ _]
                tunnel: w406 -> [w429 _]
                tunnel: [TRUE _] -> w410
                frame Default {
                  (unwired) "Folder"
                  n141 = call <resource>:"GDSProject_CreateFolder.vi"("Project Item To Create Folder Below(Use MyComputer if not wired)"=w431, "FolderName"=w425, "error in (no error)"=w430) -> ("ItemOut"=w428:refnum<vi>, "FolderCreated"=w423:bool, "error out"=w427:errorcluster)  [unwired: 13 in, 1 out]
                  n142 = case shown="True" w423 {
                    tunnel: w429 -> [_ w437]
                    tunnel: w428 -> [_ w436]
                    tunnel: w427 -> [w432 w435]
                    tunnel: [w432 w434] -> w426
                    tunnel: w425 -> [_ w433]
                    frame False {
                    }
                    frame True {
                      n143 = case shown="\"Public\", \"util\", \"utils\"" w433 {
                        tunnel: w437 -> [_ w443 w448]
                        tunnel: w436 -> [_ w442 w447]
                        tunnel: w435 -> [w438 w441 w446]
                        tunnel: [w438 w440 w445] -> w434
                        frame "Public", "util", "utils" {
                        }
                        frame "protected" {
                          n144 = invoke class="LVClassLibrary" method="Set Source Scope"(reference=w443, error in=w441, "SourceRef"=w442, "Scope"=T4."protected" ("scope")) -> (error out=w440:errorcluster)  [unwired: 1 in, 4 out]
                        }
                        frame Default {
                          n145 = invoke class="LVClassLibrary" method="Set Source Scope"(reference=w448, error in=w446, "SourceRef"=w447, "Scope"=T4."private" ("scope")) -> (error out=w445:errorcluster)  [unwired: 1 in, 4 out]
                        }
                      }
                    }
                  }
                }
                frame "" {
                }
              }
              n146 = invoke class="ProjectItem" method="AddItem"(reference=w415, error in=w418, "Name"=w405, "Path"=w409, "Type"="VI") -> (reference out=w411:refnum<vi>, error out=w404:errorcluster, "AddItem"=w403:refnum<vi>)  [unwired: 1 in, 3 out]
              n147 = Close Reference(reference=w403, error in (no error)=w404) -> ()  [unwired: 1 out]
              n148 = case shown="True" w410 {
                tunnel: w404 -> [w419 w422]
                tunnel: [w419 w421] -> w412
                tunnel: w411 -> [_ w420]
                frame False {
                }
                frame True {
                  n149 = Close Reference(reference=w420, error in (no error)=w422) -> (error out=w421:errorcluster)
                }
              }
            }
          }
          frame "CopyMemberDataControls" {
            n150 = Unbundle By Name(w502) -> ("TemplateClass"=w460:refnum<vi>, "ClassRefnum"=w453:refnum<vi>)
            n151 = invoke class="App" method="Clipboard.Empty"(error in=w462) -> (error out=w461:errorcluster)  [unwired: 2 in, 2 out]
            n152 = property class="LVClassLibrary"(reference=w460, error in=w461) -> (error out=w501:errorcluster, "Member Data"=w500:refnum<vi>)  [unwired: 1 out]
            n153 = property class="VI"(reference=w500, error in=w501, "Front Panel.Open"=FALSE ("Front Panel Window:Open")) -> (reference out=w459:refnum<vi>, error out=w497:errorcluster, "Panel"=w498:refnum<vi>)
            n154 = property class="Pnl"(reference=w498, error in=w497) -> (reference out=w494:refnum<vi>, error out=w491:errorcluster, "Controls[]"=w499:refnum<vi>[])
            n155 = Index Array(array=w499) -> (element=w495:refnum<vi>)  [unwired: 1 in]
            n156 = property class="Ctl"(reference=w495, error in=w491, "Selected"=TRUE) -> (reference out=w466:refnum<vi>, error out=w492:errorcluster)
            n157 = invoke class="Pnl" method="Copy Selection"(reference=w494, error in=w492) -> (reference out=w465:refnum<vi>, error out=w483:errorcluster)  [unwired: 1 in, 1 out]
            n158 = property class="LVClassLibrary"(reference=w453, error in=w483) -> (error out=w484:errorcluster, "Member Data"=w485:refnum<vi>)  [unwired: 1 out]
            n159 = property class="VI"(reference=w485, error in=w484, "Front Panel.Open"=FALSE ("Front Panel Window:Open")) -> (reference out=w457:refnum<vi>, error out=w488:errorcluster, "Panel"=w487:refnum<vi>)
            n160 = property class="Pnl"(reference=w487, error in=w488) -> (reference out=w479:refnum<vi>, error out=w490:errorcluster, "Controls[]"=w486:refnum<vi>[])
            n161 = Index Array(array=w486) -> (element=w489:refnum<vi>)  [unwired: 1 in]
            n162 = property class="Ctl"(reference=w489, error in=w490) -> (reference out=w481:refnum<vi>, error out=w482:errorcluster, "Position"=w473:T5)
            n163 = invoke class="Ctl" method="Delete"(reference=w481, error in=w482) -> (reference out=w472:refnum<vi>, error out=w480:errorcluster)  [unwired: 1 in, 1 out]
            n164 = Close Reference(reference=w472) -> ()  [unwired: 1 in, 1 out]
            n165 = invoke class="Pnl" method="Paste Selection"(reference=w479, error in=w480, "Pos"=T5 {"Left"=0, "Top"=0} ("Position")) -> (reference out=w476:refnum<vi>, error out=w475:errorcluster)  [unwired: 2 in, 3 out]
            n166 = property class="Pnl"(reference=w476, error in=w475) -> (reference out=w470:refnum<vi>, error out=w474:errorcluster, "Controls[]"=w478:refnum<vi>[])
            n167 = Index Array(array=w478) -> (element=w477:refnum<vi>)  [unwired: 1 in]
            n168 = property class="Ctl"(reference=w477, error in=w474, "Position"=w473) -> (reference out=w471:refnum<vi>, error out=w467:errorcluster)
            n169 = Close Reference(reference=w471, error in (no error)=w467) -> (error out=w496:errorcluster)
            n170 = Close Reference(reference=w470, error in (no error)=w496) -> (error out=w458:errorcluster)
            n171 = invoke class="VI" method="Save.Instrument"(reference=w457, error in=w458) -> (error out=w455:errorcluster)  [unwired: 4 in, 5 out]
            n172 = invoke class="LVClassLibrary" method="Save"(reference=w453, error in=w455) -> (error out=w454:errorcluster)  [unwired: 2 in, 3 out]
            n173 = Close Reference(reference=w457, error in (no error)=w454) -> (error out=w452:errorcluster)
            n174 = Close Reference(reference=w466, error in (no error)=w452) -> (error out=w468:errorcluster)
            n175 = Close Reference(reference=w465, error in (no error)=w468) -> (error out=w469:errorcluster)
            n176 = Close Reference(reference=w459, error in (no error)=w469) -> (error out=w451:errorcluster)
            n177 = invoke class="App" method="Clipboard.Empty"(error in=w451) -> ()  [unwired: 2 in, 3 out]
          }
          frame "UpdateIcons" {
            n178 = Unbundle By Name(w517) -> ("ClassRefnum"=w516:refnum<vi>)
            n179 = Unbundle By Name(w517) -> ("SubClass"=w521:bool, "ClassName"=w518:string)
            n180 = call-dynamic "ProgressWindow.vi"("ClassWriter in"=w504, "Message(Exit)"="Hide", "error in (no error)"=w508) -> ("ClassWriter out"=w510:refnum<class "ClassWriterNative.lvclass">, "error out"=w507:errorcluster)  [unwired: 15 in]
            n181 = Empty String/Path?(string/path=w513) -> (empty?=w514:bool)
            n182 = Not(x=w514) -> (.not. x?=w512:bool)
            n183 = call <resource>:"GDSLvIcon_DialogUpdateClass.vi"("ClassPath(FilePath/ProjectTreePath/LvCLassRef)"=w516, "ClassName"=w518, "AutoUpdate"=w512, "error in (no error)"=w507, "HeaderToApply (take from VIRef or /use 2D-8bit header, Ignored if not wired)"=w513) -> ("error out"=w506:errorcluster)  [unwired: 14 in]
            n184 = Select(t="ReplaceBaseTemplateReferences", s=w521, f="AddFolders") -> (s? t:f=w519:string)
            n185 = call-dynamic "ProgressWindow.vi"("ClassWriter in"=w510, "Message(Exit)"="UnHide", "error in (no error)"=w506) -> ("error out"=w505:errorcluster)  [unwired: 15 in, 1 out]
          }
          frame "ReplaceBaseTemplateReferences" {
            # "This is a sub class, replace all BaseClass References with Select base class.\nIf base not equal to root, also replace BaseClass ObjectRef with Root-Base ObjectRef"
            n186 = Unbundle By Name(w536) -> ("VIs"=w541:refnum<vi>[], "TemplateClass"=w525:refnum<vi>, "BaseClassFolder"=w535:path, "BaseClassName"=w538:string)
            n187 = Unbundle By Name(w536) -> ()  [unwired: 1 out]
            n188 = property class="LVClassLibrary"(reference=w525) -> ("Parent"=w524:refnum<vi>)  [unwired: 1 in, 2 out]
            n189 = property class="LVClassLibrary"(reference=w524) -> (reference out=w522:refnum<vi>, error out=w523:errorcluster, "Name"=w528:string)  [unwired: 1 in]
            n190 = Format Into String(LvNativeTemplateNames."NativeBaseTemplate" ("TemplateNames")) -> ()  [unwired: 3 in, 2 out]
            n191 = Close Reference(reference=w522, error in (no error)=w523) -> ()  [unwired: 1 out]
            n192 = Match Pattern(string=w528, regular expression="\\2E[Ll][Vv][Cc][Ll][Aa][Ss][Ss]$") -> (before substring=w526:string)  [unwired: 1 in, 3 out]
            n193 = call-dynamic "GetTemplatePath.vi"("reference in"=w531, "ClassTemplateSubDirectory"=w526, "error in (no error)"=w529) -> ("FolderPathOut"=w537:path, "error out"=w530:errorcluster)  [unwired: 12 in, 3 out]
            n194 = call <resource>:"GOOP300_FindFilesToExchange.vi"("OldClassName(Prefix or suffix for some VIs)"=w526, "OldFolderPath"=w537, "NewFolderPath"=w535, "NewClassName(Prefix or suffix for some VIs)"=w538) -> ("OldFiles"=w533:path[], "NewFileArray"=w532:path[])  [unwired: 14 in]
            n195 = for {
              tunnel: w541 -> [w546] mode=indexing
              shift-right: [w544] -> w540
              shift-left: w530 -> [w545]
              tunnel: w533 -> [w543]
              tunnel: w532 -> [w542]
              n196 = call <resource>:"Scripting_ReplaceVisAndControls.vi"("ViRef"=w546, "OldVIsAndControls"=w543, "NewVIsAndControls"=w542, "error in (no error)"=w545) -> ("error out"=w544:errorcluster)  [unwired: 14 in, 1 out]
            }
          }
          frame "AddFolders" {
            n197 = Unbundle By Name(w557) -> ("ClassRefnum"=w556:refnum<vi>)
            n198 = call <resource>:"GDSProject_CreateFolder.vi"("Project Item To Create Folder Below(Use MyComputer if not wired)"=w556, "FolderName"="private", "error in (no error)"=w555, "CreateThePhysicalFolderIfPossible(False)"=TRUE ("CreateThePfysicalFolderIfPossible(False)")) -> ("ItemOut"=w562:refnum<vi>, "error out"=w560:errorcluster)  [unwired: 12 in, 2 out]
            n199 = invoke class="LVClassLibrary" method="Set Source Scope"(reference=w556, error in=w560, "SourceRef"=w562, "Scope"=T4."private" ("scope")) -> (reference out=w547:refnum<vi>, error out=w550:errorcluster)  [unwired: 1 in, 3 out]
            n200 = call <resource>:"GDSProject_CreateFolder.vi"("Project Item To Create Folder Below(Use MyComputer if not wired)"=w547, "FolderName"="protected", "error in (no error)"=w550, "CreateThePhysicalFolderIfPossible(False)"=TRUE ("CreateThePfysicalFolderIfPossible(False)")) -> ("ItemOut"=w552:refnum<vi>, "error out"=w553:errorcluster)  [unwired: 12 in, 2 out]
            n201 = invoke class="LVClassLibrary" method="Set Source Scope"(reference=w547, error in=w553, "SourceRef"=w552, "Scope"=T4."protected" ("scope")) -> (error out=w549:errorcluster)  [unwired: 1 in, 4 out]
          }
          frame "SetClassProperties" {
            n202 = Unbundle By Name(w587) -> ("ClassDescription"=w583:string)
            n203 = Unbundle By Name(w566) -> ("ClassRefnum"=w574:refnum<vi>)
            n204 = Unbundle By Name(w566) -> ("TemplateName"=w582:string, "SubClass"=w592:bool)
            n205 = Unbundle By Name(w566) -> ("BaseClassFolder"=w591:path)
            n206 = Unbundle By Name(w566) -> ("TemplateClass"=w581:refnum<vi>)
            n207 = case shown="True" w592 {
              tunnel: w574 -> [w599 w609]
              tunnel: [w599 w608] -> w589
              tunnel: w573 -> [w596 w606]
              tunnel: [w595 w605] -> w588
              tunnel: w591 -> [_ w607]
              tunnel: [w594 w601] -> w567
              frame False {
                n208 = call <resource>:"BaseProvider_ConfigurationMemory.vi"("error in (no error)"=w596, "Action"=enum16{"Read", "Load", "Save"}."Read") -> ("PatternOut"=w598:T11, "error out"=w595:errorcluster)  [unwired: 11 in, 5 out]
                n209 = Format Into String(w598) -> (resulting string=w594:string)  [unwired: 3 in, 1 out]
              }
              frame True {
                n210 = call <resource>:"GDSProject_OpenClass.vi"("ClassPath(FilePath/ProjectTreePath/LvCLassRef)"=w607, "error IO"=w606) -> ("LVClass.Open"=w604:refnum<vi>, "error out"=w603:errorcluster)  [unwired: 15 in, 1 out]
                n211 = call <resource>:"GDSLvClass_ReadClassType.vi"("Class Refnum In"=w604) -> ("Class Refnum Out"=w602:refnum<vi>, "ClassSettings"=w600:T7)  [unwired: 16 in, 1 out]
                n212 = property class="LVClassLibrary"(reference=w609, error in=w603, "Parent"=w602) -> (reference out=w608:refnum<vi>, error out=w605:errorcluster)
                n213 = Unbundle By Name(w600) -> ("ConnectorPanePattern"=w601:string)
                n214 = Close Reference(reference=w602, error in (no error)=w605) -> ()  [unwired: 1 out]
              }
            }
            n215 = property class="LVClassLibrary"(reference=w581) -> ("Version"=w580:T12)  [unwired: 1 in, 2 out]
            n216 = Unbundle(w580) -> ("Major"=w578:u16, "Minor"=w577:u16, "Fix"=w576:u16, "Build"=w575:u16)
            n217 = Format Into String(format string="%d.%d.%d.%d", w578, w577, w576, w575) -> (resulting string=w564:string)  [unwired: 2 in, 1 out]
            n218 = Format Into String(LvNativeProviderName."Endevo LabVIEW Native" ("ProviderName")) -> (resulting string=w584:string)  [unwired: 3 in, 1 out]
            n219 = Bundle By Name(cluster=T7 {"ClassProviderName"="", "ClassTemplateUsed"="", "ClassTemplateVersion"="", "ClassDescription"="", "PlugIns"=[], "ConnectorPanePattern"=""} ("ClassSettings"), "ClassProviderName"=w584, "ClassTemplateUsed"=w582, "ClassTemplateVersion"=w564, "ClassDescription"=w583, "ConnectorPanePattern"=w567) -> (w585:T7)
            n220 = Bundle By Name(cluster=w566, "TemplateVersionUsed"=w564) -> (w565:T2)
            n221 = call <resource>:"GDSLvClass_StoreClassType.vi"("Class Refnum In"=w589, "ClassSettings"=w585, "error in (no error)"=w588) -> ("Class Refnum Out"=w571:refnum<vi>, "error out"=w570:errorcluster)  [unwired: 15 in]
            n222 = call <resource>:"UpdateClassApperance.vi"("ClassRefIn"=w571, "error in (no error)"=w570) -> ("ClassRefOut"=w569:refnum<vi>, "error out"=w568:errorcluster)  [unwired: 16 in]
            n223 = invoke class="LVClassLibrary" method="Save"(reference=w569, error in=w568) -> (error out=w590:errorcluster)  [unwired: 2 in, 3 out]
          }
          frame "FixAttribute" {
            w638 = refnum<vi> refnum  # Control
            w642 = refnum<vi> refnum  # Cluster
            # "JUST BECASUSE IT FAILS SOMETIMES"
            n224 = Unbundle By Name(w644) -> ("ClassRefnum"=w621:refnum<vi>)
            n225 = property class="LVClassLibrary"(reference=w621, error in=w622) -> (error out=w650:errorcluster, "Member Data"=w613:refnum<vi>)  [unwired: 1 out]
            n226 = property class="VI"(reference=w613, error in=w650, "Front Panel.Open"=FALSE ("Front Panel Window:Open")) -> (error out=w618:errorcluster, "Panel"=w648:refnum<vi>)  [unwired: 1 out]
            n227 = property class="Pnl"(reference=w648, error in=w618) -> (reference out=w626:refnum<vi>, error out=w633:errorcluster, "Controls[]"=w649:refnum<vi>[])
            n228 = Index Array(array=w649) -> (element=w643:refnum<vi>)  [unwired: 1 in]
            n229 = To More Specific Class(target class=w642, reference=w643, error in=w633) -> (specific class reference=w641:refnum<vi>, error out=w634:errorcluster)
            n230 = property class="Clust"(reference=w641, error in=w634) -> (reference out=w628:refnum<vi>, error out=w635:errorcluster, "AllObjs[]"=w640:refnum<vi>[])
            n231 = Index Array(array=w640) -> (element=w639:refnum<vi>)  [unwired: 1 in]
            n232 = To More Specific Class(target class=w638, reference=w639, error in=w635) -> (specific class reference=w637:refnum<vi>, error out=w636:errorcluster)
            n233 = property class="Ctl"(reference=w637, error in=w636) -> (reference out=w632:refnum<vi>, error out=w631:errorcluster, "Label.Text"=w630:string, "Label.Left"=w611:i32)
            n234 = disable-structure shown="Enabled" {
              disable-tunnel: w632 -> [w658 w659]
              disable-tunnel: w631 -> [w656 w660]
              disable-tunnel: [w655 w659] -> w620
              disable-tunnel: [w653 w660] -> w619
              disable-tunnel: w613 -> [w652 _]
              frame Disabled {
                n235 = property class="Ctl"(reference=w658, error in=w656, "Label.Text"="UpdateMe") -> (reference out=w655:refnum<vi>, error out=w654:errorcluster)
                n236 = invoke class="VI" method="Save.Instrument"(reference=w652, error in=w654) -> (error out=w653:errorcluster)  [unwired: 4 in, 5 out]
              }
              frame Enabled {
              }
            }
            n237 = Increment(x=w611) -> (x+1=w610:i32)
            n238 = property class="Ctl"(reference=w620, error in=w619, "Label.Text"=w630, "Label.Left"=w610) -> (reference out=w615:refnum<vi>, error out=w629:errorcluster)
            n239 = Close Reference(reference=w615, error in (no error)=w629) -> (error out=w614:errorcluster)
            n240 = invoke class="VI" method="Save.Instrument"(reference=w613, error in=w614) -> (error out=w612:errorcluster)  [unwired: 4 in, 5 out]
            n241 = invoke class="VI" method="CtlVIApplyChanges"(reference=w613, error in=w612) -> (reference out=w617:refnum<vi>, error out=w616:errorcluster)  [unwired: 1 in, 1 out]
            n242 = Close Reference(reference=w628, error in (no error)=w616) -> (error out=w627:errorcluster)
            n243 = Close Reference(reference=w626, error in (no error)=w627) -> (error out=w625:errorcluster)
            n244 = invoke class="VI" method="Save.Instrument"(reference=w617, error in=w625) -> (reference out=w624:refnum<vi>, error out=w646:errorcluster)  [unwired: 4 in, 4 out]
            n245 = invoke class="LVClassLibrary" method="Save"(reference=w621, error in=w646) -> (error out=w645:errorcluster)  [unwired: 2 in, 3 out]
            n246 = Close Reference(reference=w624, error in (no error)=w645) -> (error out=w623:errorcluster)
          }
          frame "CloseRefs", "Error", Default {
            n247 = case shown="Default" w669 {
              tunnel: w675 -> [w683 w690]
              tunnel: w666 -> [w682 w691]
              tunnel: [w681 w690] -> w665
              frame "CloseRefs" {
                n248 = Unbundle By Name(w682) -> ("VIs"=w684:refnum<vi>[])
                n249 = for {
                  tunnel: w684 -> [w687] mode=indexing
                  shift-right: [w689] -> w681
                  shift-left: w683 -> [w688]
                  n250 = invoke class="VI" method="Save.Instrument"(reference=w687, error in=w688) -> (reference out=w685:refnum<vi>, error out=w686:errorcluster)  [unwired: 4 in, 4 out]
                  n251 = Close Reference(reference=w685, error in (no error)=w686) -> (error out=w689:errorcluster)
                }
              }
              frame Default {
                n252 = Unbundle By Name(w691) -> ("VIs"=w692:refnum<vi>[])
                n253 = for {
                  tunnel: w692 -> [w693] mode=indexing
                  n254 = Close Reference(reference=w693) -> ()  [unwired: 1 in, 1 out]
                }
              }
            }
            n255 = Unbundle By Name(w666) -> ("App"=w661:refnum<vi>, "TemplateClass"=w674:refnum<vi>, "ProjectRefnum"=w671:refnum<vi>, "ClassRefnum"=w670:refnum<vi>)
            n256 = case shown="False" w664 {
              tunnel: [w679 w680] -> w673
              tunnel: w670 -> [w678 _]
              tunnel: w665 -> [w677 w680]
              frame False {
                n257 = Close Reference(reference=w678, error in (no error)=w677) -> (error out=w679:errorcluster)
              }
              frame True {
              }
            }
            n258 = Close Reference(reference=w671, error in (no error)=w673) -> (error out=w672:errorcluster)
            n259 = Close Reference(reference=w674, error in (no error)=w672) -> (error out=w663:errorcluster)
            n260 = Close Reference(reference=w661, error in (no error)=w663) -> (error out=w662:errorcluster)
            n261 = call <resource>:"GDSError_LogErrorInformation.vi"("State"=w667, "LocalVariableData"=w666, "error in (no error)"=w662) -> ("error out"=w668:errorcluster)  [unwired: 16 in]
          }
        }
        n262 = Equal?(x=w31, y="Exit") -> (x = y?=w35:bool)
        n263 = Select(t="Error", s=w30, f=w31) -> (s? t:f=w34:string)
      }
    }
    frame Error {
    }
  }
  "error out" <- w7
  n264 = Unbundle By Name(w3) -> ("ClassRefnum"=→"LVClassLibraryRefnum":refnum<vi>, "TemplateVersionUsed"=→"TemplateVersionUsed":string)
  "ClassWriterNative" <- "ClassWriterNative"
